vi "generate linear region.vi"(7 "number of  grid points":i32, 10 "center":dbl, 11 "delta":dbl) -> (3 "real axis":dbl[](array[numeric])=[-0.001573233, -0.0015680711305333334, -0.0015629092610666667, -0.0015577473916, -0.0015525855221333333, -0.0015474236526666666, -0.0015422617832000001, -0.0015370999137333335, -0.0015319380442666668, -0.0015267761748, -0.0015216143053333334, -0.0015164524358666667, -0.0015112905664, -0.0015061286969333333, -0.0015009668274666666, -0.001495804958, -0.0014906430885333333, -0.0014854812190666668, -0.0014803193496000001, -0.0014751574801333334, -0.0014699956106666667, -0.0014648337412, -0.0014596718717333334, -0.0014545100022666667, -0.0014493481328, -0.0014441862633333333, -0.0014390243938666668, -0.0014338625244000001, -0.0014287006549333335, -0.0014235387854666668, -0.001418376916, -0.0014132150465333334, -0.0014080531770666667, -0.0014028913076, -0.0013977294381333333, -0.0013925675686666666, -0.0013874056992, -0.0013822438297333333, -0.0013770819602666666, -0.0013719200908000001, -0.0013667582213333334, -0.0013615963518666667, -0.0013564344824, -0.0013512726129333334, -0.0013461107434666667, -0.001340948874, -0.0013357870045333333, -0.0013306251350666666, -0.0013254632656000001, -0.0013203013961333335, -0.0013151395266666668, -0.0013099776572, -0.0013048157877333334, -0.0012996539182666667, -0.0012944920488, -0.0012893301793333333, -0.0012841683098666666, -0.0012790064404, -0.0012738445709333333, -0.0012686827014666666, -0.001263520832, -0.0012583589625333334, -0.0012531970930666667, -0.0012480352236, -0.0012428733541333334, -0.0012377114846666667, -0.0012325496152, -0.0012273877457333333, -0.0012222258762666668, -0.0012170640068000001, -0.0012119021373333335, -0.0012067402678666668, -0.0012015783984, -0.0011964165289333334, -0.0011912546594666667, -0.00118609279, -0.0011809309205333333, -0.0011757690510666666, -0.0011706071816, -0.0011654453121333333, -0.0011602834426666666, -0.0011551215731999999, -0.0011499597037333334, -0.0011447978342666667, -0.0011396359648, -0.0011344740953333334, -0.0011293122258666667, -0.0011241503564, -0.0011189884869333333, -0.0011138266174666666, -0.0011086647480000001, -0.0011035028785333334, -0.0010983410090666668, -0.0010931791396, -0.0010880172701333334, -0.0010828554006666667, -0.0010776935312, -0.0010725316617333333, -0.0010673697922666666, -0.0010622079228, -0.0010570460533333333, -0.0010518841838666666, -0.0010467223143999999, -0.0010415604449333332, -0.0010363985754666667, -0.001031236706, -0.0010260748365333334, -0.0010209129670666667, -0.0010157510976, -0.0010105892281333333, -0.0010054273586666668, -0.0010002654892000001, -0.0009951036197333334, -0.0009899417502666668, -0.0009847798808, -0.0009796180113333334, -0.0009744561418666667, -0.0009692942724, -0.0009641324029333333, -0.0009589705334666666, -0.000953808664, -0.0009486467945333334, -0.0009434849250666667, -0.0009383230556, -0.0009331611861333333, -0.0009279993166666666, -0.0009228374472, -0.0009176755777333334, -0.0009125137082666667, -0.0009073518388, -0.0009021899693333333, -0.0008970280998666667, -0.0008918662304, -0.0008867043609333333, -0.0008815424914666666, -0.000876380622, -0.0008712187525333334, -0.0008660568830666667, -0.0008608950136, -0.0008557331441333333, -0.0008505712746666666, -0.0008454094052, -0.0008402475357333334, -0.0008350856662666667, -0.0008299237968, -0.0008247619273333333, -0.0008196000578666666, -0.0008144381884, -0.0008092763189333334, -0.0008041144494666667, -0.00079895258, -0.0007937907105333333, -0.0007886288410666666, -0.0007834669716, -0.0007783051021333333, -0.0007731432326666666, -0.0007679813632, -0.0007628194937333333, -0.0007576576242666667, -0.0007524957548, -0.0007473338853333333, -0.0007421720158666666, -0.0007370101463999999, -0.0007318482769333334, -0.0007266864074666667, -0.000721524538, -0.0007163626685333333, -0.0007112007990666666, -0.0007060389296, -0.0007008770601333333, -0.0006957151906666667, -0.0006905533212, -0.0006853914517333333, -0.0006802295822666666, -0.0006750677128, -0.0006699058433333333, -0.0006647439738666666, -0.0006595821044, -0.0006544202349333333, -0.0006492583654666667, -0.000644096496, -0.0006389346265333333, -0.0006337727570666666, -0.0006286108875999999, -0.0006234490181333333, -0.0006182871486666667, -0.0006131252792, -0.0006079634097333333, -0.0006028015402666666, -0.0005976396707999999, -0.0005924778013333333, -0.0005873159318666667, -0.0005821540624, -0.0005769921929333333, -0.0005718303234666666, -0.0005666684539999999, -0.0005615065845333332, -0.0005563447150666665, -0.0005511828456000001, -0.0005460209761333334, -0.0005408591066666667, -0.0005356972372, -0.0005305353677333333, -0.0005253734982666666, -0.0005202116287999999, -0.0005150497593333333, -0.0005098878898666666, -0.0005047260203999999, -0.0004995641509333334, -0.0004944022814666667, -0.000489240412, -0.00048407854253333335, -0.00047891667306666666, -0.00047375480359999997, -0.0004685929341333333, -0.0004634310646666666, -0.0004582691951999999, -0.0004531073257333332, -0.00044794545626666653, -0.00044278358680000006, -0.0004376217173333334, -0.0004324598478666667, -0.0004272979784, -0.0004221361089333333, -0.0004169742394666666, -0.00041181236999999994, -0.00040665050053333325, -0.00040148863106666656, -0.0003963267615999999, -0.0003911648921333332, -0.0003860030226666667, -0.00038084115320000003, -0.00037567928373333334, -0.00037051741426666666, -0.00036535554479999997, -0.0003601936753333333, -0.0003550318058666666, -0.0003498699363999999, -0.0003447080669333332, -0.00033954619746666653, -0.00033438432799999984, -0.0003292224585333334, -0.0003240605890666667, -0.0003188987196, -0.0003137368501333333, -0.0003085749806666666, -0.00030341311119999994, -0.00029825124173333325, -0.00029308937226666656, -0.0002879275027999999, -0.0002827656333333332, -0.0002776037638666667, -0.00027244189440000003, -0.00026728002493333334, -0.00026211815546666665, -0.00025695628599999997, -0.0002517944165333333, -0.0002466325470666666, -0.0002414706775999999, -0.00023630880813333322, -0.00023114693866666653, -0.00022598506919999984, -0.00022082319973333337, -0.00021566133026666668, -0.0002104994608, -0.0002053375913333333, -0.00020017572186666662, -0.00019501385239999993, -0.00018985198293333325, -0.00018469011346666656, -0.00017952824399999987, -0.00017436637453333318, -0.00016920450506666671, -0.00016404263560000003, -0.00015888076613333334, -0.00015371889666666665, -0.00014855702719999996, -0.00014339515773333328, -0.0001382332882666666, -0.0001330714187999999, -0.00012790954933333321, -0.00012274767986666653, -0.00011758581039999984, -0.00011242394093333337, -0.00010726207146666668, -0.000102100202, -9.69383325333333e-05, -9.177646306666662e-05, -8.661459359999993e-05, -8.145272413333324e-05, -7.629085466666656e-05, -7.112898519999987e-05, -6.596711573333318e-05, -6.0805246266666495e-05, -5.5643376800000024e-05, -5.048150733333334e-05, -4.531963786666665e-05, -4.015776839999996e-05, -3.4995898933333274e-05, -2.9834029466666587e-05])   [LabVIEW 2018]
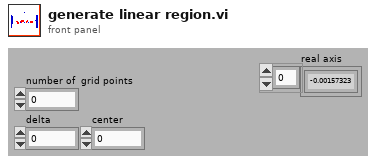
[diagram p1: front panel]
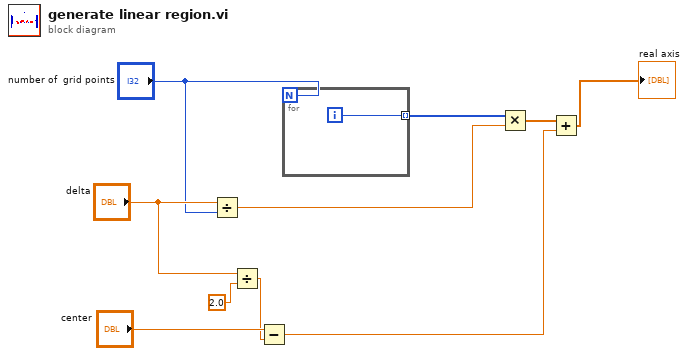
[diagram p0: block diagram]
diagram:
  n1 = Divide(x="delta", y="number of  grid points") -> (x/y=w3:dbl)
  n2 = Divide(x="delta", y=2.0) -> (x/y=w7:dbl)
  n3 = Subtract(x="center", y=w7) -> (x-y=w4:dbl)
  n4 = for {
    N: "number of  grid points" -> [_]
    tunnel: [w11] -> w2 mode=indexing
    i -> [w11]
  }
  n5 = Multiply(x=w2, y=w3) -> (x*y=w6:dbl[])
  n6 = Add(x=w6, y=w4) -> (x+y=→"real axis":dbl[])
